vi "Configured.vi"(8 "error in (no error)":errorcluster, 11 "Device in":refnum<class "Device.lvclass">) -> (0 "error out":errorcluster, 2 "Configured":bool, 3 "Device out":refnum<class "Device.lvclass">)   [LabVIEW 2015, in "IBEX Device.lvlib" / "Device.lvclass"]
doc: "Indicates that the Device is configured and is ready to be used."
uses:
  Device.lvclass
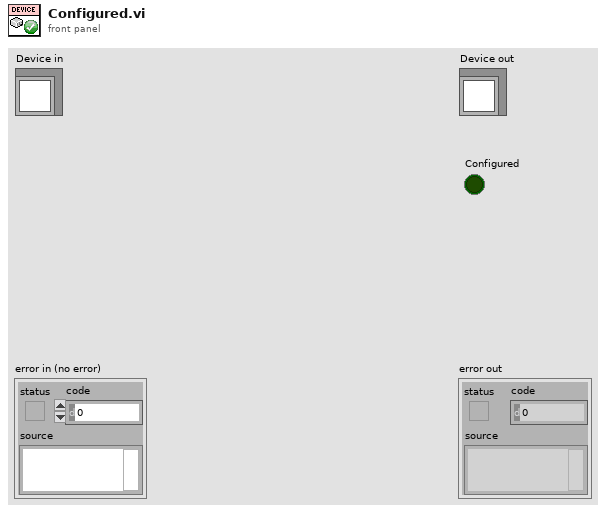
[diagram p1: front panel]
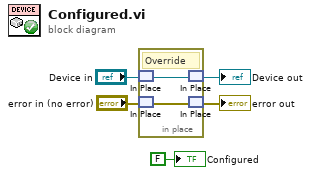
[diagram p0: block diagram]
diagram:
  n1 = in-place {
    # "Override"
    n2 = in-place-match #1("Device in") -> (w7:refnum<class "Device.lvclass">)
    n3 = in-place-match #2("error in (no error)") -> (w6:errorcluster)
    n4 = in-place-match #1(w7) -> (→"Device out":refnum<class "Device.lvclass">)
    n5 = in-place-match #2(w6) -> (→"error out":errorcluster)
  }
  "Configured" <- FALSE ("Configured")
